vi "FlashWindow.vi"(8 "No Error":errorcluster, 10 "Flash Operation":T1, 11 "Window [SDL_Window *]":i64) -> (0 "error out":errorcluster)   [LabVIEW 2024, in "SDL3.lvlib" / "Video.lvlib"]
doc: "<B>Summary</B>\nRequest a window to demand attention from the user."
uses:
  Video.lvlib
  FlashOperation--enum.ctl
  Error/Error.lvlib
  Lib/SDL3-32.dll
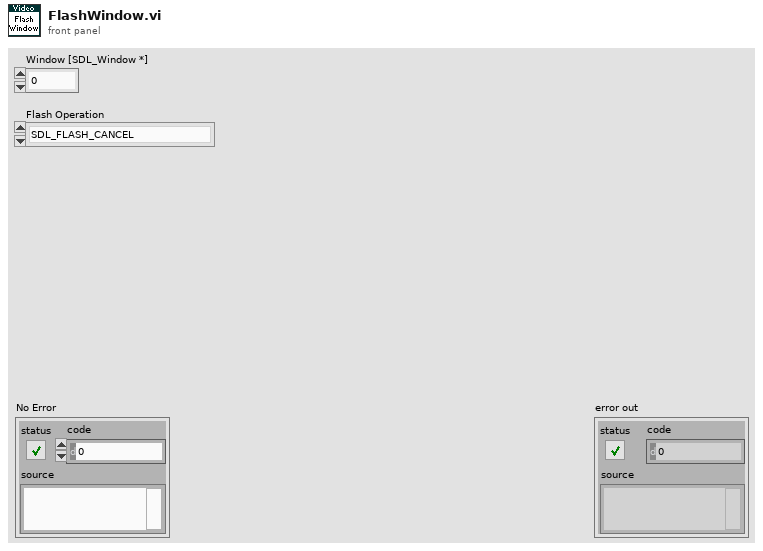
[diagram p1: front panel]
types:
  T1 = typedef "SDL3.lvlib/Video.lvlib/FlashOperation--enum.ctl" = enum32{"SDL_FLASH_CANCEL", "SDL_FLASH_BRIEFLY", "SDL_FLASH_UNTIL_FOCUSED"}
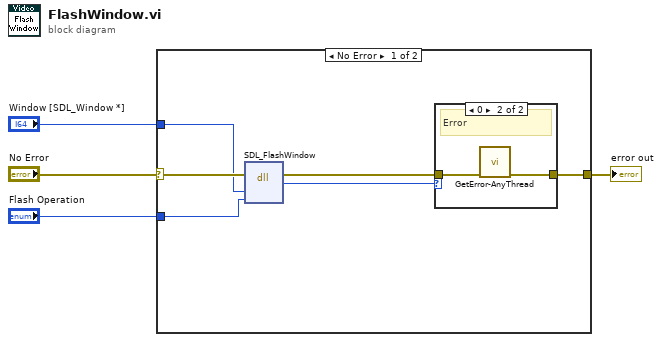
[diagram p0: block diagram]
diagram:
  n1 = case shown="No Error" "No Error" {
    selector: "No Error" -> [w10 w14]
    tunnel: [w7 w14] -> w3
    tunnel: "Window [SDL_Window *]" -> [w9 _]
    tunnel: "Flash Operation" -> [w5 _]
    frame No Error {
      n2 = dll-call lib="C:/Users/Thomas/Documents/Projects/LV-SDL3/Lib/SDL3-*.*" fn="SDL_FlashWindow"(error in=w10, "window"=w9, "operation"=w5) -> (error out=w8:errorcluster, "return type"=w6:i32)  [unwired: 4 in, 1 out]
      n3 = case shown="0" w6 {
        tunnel: w8 -> [w11 w13]
        tunnel: [w11 w12] -> w7
        frame Default {
          # "Ok"
        }
        frame 0 {
          # "Error"
          n4 = call "GetError-AnyThread.vi"("No Error"=w13) -> ("error out"=w12:errorcluster)  [unwired: 10 in]
        }
      }
    }
    frame Error {
    }
  }
  "error out" <- w3
